vi "Call Keep ApplyLib in Memory.vi"   [LabVIEW 2020]
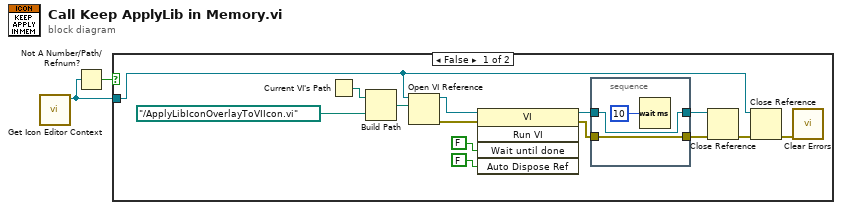
[diagram p0: block diagram]
diagram:
  n1 = call "Get Icon Editor Context.vi"() -> ("icon editor context"=w2:refnum<vi>)  [unwired: 11 in]
  n2 = Not A Number/Path/Refnum?(number/path/refnum=w2) -> (NaN/Path/Refnum?=w1:bool)
  n3 = case shown="False" w1 {
    tunnel: w2 -> [w6 _]
    frame False {
      n4 = Current VI's Path() -> (path=w3:path)
      n5 = Build Path(base path=w3, name or relative path=path "../ApplyLibIconOverlayToVIIcon.vi") -> (appended path=w14:path)
      n6 = Open VI Reference(application reference (local)=w6, vi path=w14) -> (vi reference=w13:refnum<vi>, error out=w12:errorcluster)  [unwired: 1 in, 3 out]
      n7 = invoke class="VI" method="Run VI"(reference=w13, error in=w12, "Wait until done"=FALSE ("Wait Until Done"), "Auto Dispose Ref"=FALSE ("Auto Dispose Reference")) -> (reference out=w10:refnum<vi>, error out=w11:errorcluster)  [unwired: 1 in, 3 out]
      n8 = stacked-sequence {
        tunnel: w11 -> [w17]
        tunnel: [w18] -> w9
        tunnel: w10 -> [w18]
        tunnel: [w17] -> w8
        frame #0 {
          n9 = Wait (ms)(milliseconds to wait=u32 10) -> ()  [unwired: 1 out]
        }
      }
      n10 = Close Reference(reference=w9, error in (no error)=w8) -> (error out=w7:errorcluster)
      n11 = Close Reference(reference=w6, error in (no error)=w7) -> (error out=w5:errorcluster)
      n12 = call <vilib>:"Clear Errors.vi"("error in (no error)"=w5) -> ()  [unwired: 5 in, 2 out]
    }
    frame True {
    }
  }
